vi "lookup speed test.vi"() -> ()   [LabVIEW 2013, in "tag bus tests.lvlib"]
uses:
  tag bus tests.lvlib
  dictionary/data bus dictionary.lvclass
panel:
  out "ok":bool
  out "found":bool[](array[boolean])
  out "x-y":dbl
  in  "count":i32=5000
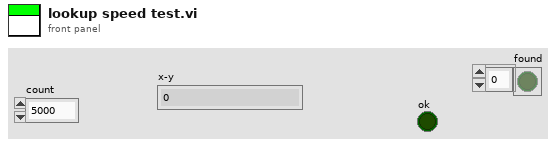
[diagram p1: front panel]
types:
  T1 = typedef "data bus tag description.lvclass/Data Type.ctl" = enum16{"Double", "I64", "Boolean", "Array of Double", "Array of I64", "Variant"}
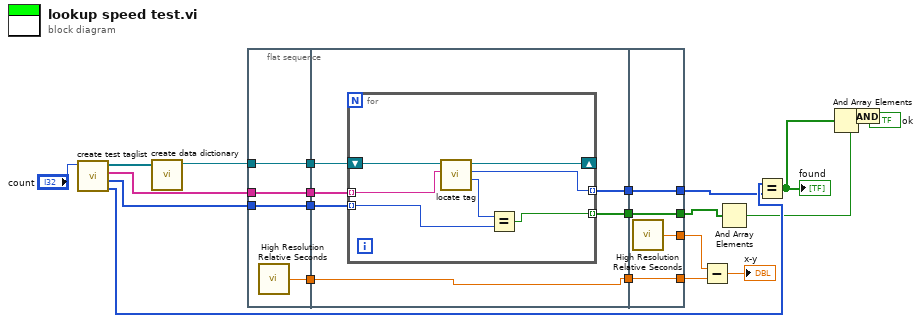
[diagram p0: block diagram]
diagram:
  n1 = call "create test taglist.vi"("count"="count") -> ("indices"=w9:i32[], "types"=w10:T1[], "names/metadata"=w12:string[], "tags"=w21:refnum<class "data bus tag description.lvclass">[])  [unwired: 7 in]
  n2 = call "create data dictionary.vi"("system tags"=w21) -> ("data dictionary"=w14:refnum<class "data bus dictionary.lvclass">)  [unwired: 9 in, 1 out]
  n3 = flat-sequence {
    tunnel: [w26] -> w17
    tunnel: [w25] -> w15
    tunnel: w14 -> [w25]
    tunnel: [w24] -> w13
    tunnel: w12 -> [w24]
    tunnel: [w23] -> w11
    tunnel: w10 -> [w23]
    tunnel: [w32] -> w19
    tunnel: w17 -> [w32]
    tunnel: w15 -> [w31]
    tunnel: w13 -> [w30]
    tunnel: w11 -> [w29]
    tunnel: [w28] -> w7
    tunnel: [w27] -> w4
    tunnel: [w43] -> w20
    tunnel: w19 -> [w42]
    tunnel: [w42] -> w18
    tunnel: [w41] -> w8
    tunnel: w7 -> [w41]
    tunnel: [w40] -> w3
    tunnel: w4 -> [w40]
    frame #0 {
      n4 = call <vilib>:"High Resolution Relative Seconds.vi"() -> ("relative seconds"=w26:dbl)
    }
    frame #1 {
      n5 = for {
        shift-right: [w38] -> _
        shift-left: w31 -> [w39]
        tunnel: w30 -> [w37] mode=indexing
        tunnel: w29 -> [w34] mode=indexing
        tunnel: [w36] -> w28 mode=indexing
        tunnel: [w33] -> w27 mode=indexing
        n6 = call "locate tag.vi"("name"=w37, "data dictionary in"=w39) -> ("data type"=w35:T1, "index"=w36:i32, "data dictionary out"=w38:refnum<class "data bus dictionary.lvclass">)  [unwired: 6 in, 1 out]
        n7 = Equal?(x=w35, y=w34) -> (x = y?=w33:bool)
      }
    }
    frame #2 {
      n8 = call <vilib>:"High Resolution Relative Seconds.vi"() -> ("relative seconds"=w43:dbl)
    }
  }
  n9 = Subtract(x=w20, y=w18) -> (x-y=→"x-y":dbl)
  n10 = And Array Elements(Boolean array=w3) -> (logical AND=w1:bool)
  n11 = Equal?(x=w9, y=w8) -> (x = y?=w6:bool[])
  "found" <- w6
  n12 = And Array Elements(Boolean array=w6) -> (logical AND=w5:bool)
  n13 = And(x=w1, y=w5) -> (x .and. y?=→"ok":bool)
